vi "Auxiliary_data_to_file.vi"(2 "error in":errorcluster, 3 "Auxiliary Data":T1 {"EOS" items=["Ideal", "CH4_van_der_Waal", "CH4_Redlich_Kwong", "CO2_van_der_Waal", "CO2_Redlich_Kwong", ""]}, 4 "Byte Stream File in":refnum<file>) -> (0 "error out":errorcluster, 1 "Byte Stream File out":refnum<file>)   [LabVIEW 2016]
uses:
  auxiliary_cluster.ctl
  EOS.ctl
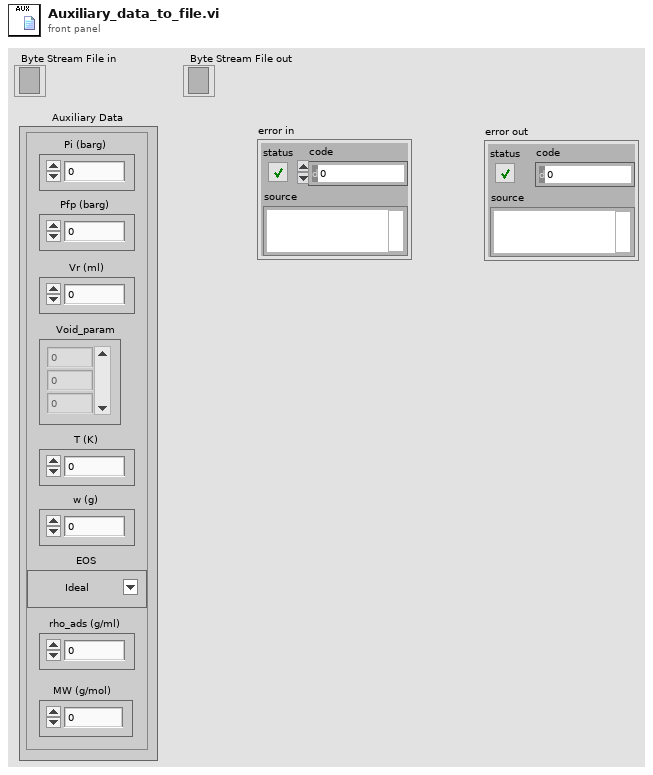
[diagram p1: front panel]
types:
  T1 = typedef "auxiliary_cluster.ctl" = cluster{"Pi (barg)":dbl, "Pfp (barg)":dbl, "Vr (ml)":dbl, "T (K)":dbl, "w (g)":dbl, "Void_param":dbl[], "EOS":T2, "rho_ads (g/ml)":dbl, "MW (g/mol)":dbl}
  T2 = typedef "EOS.ctl" = u16
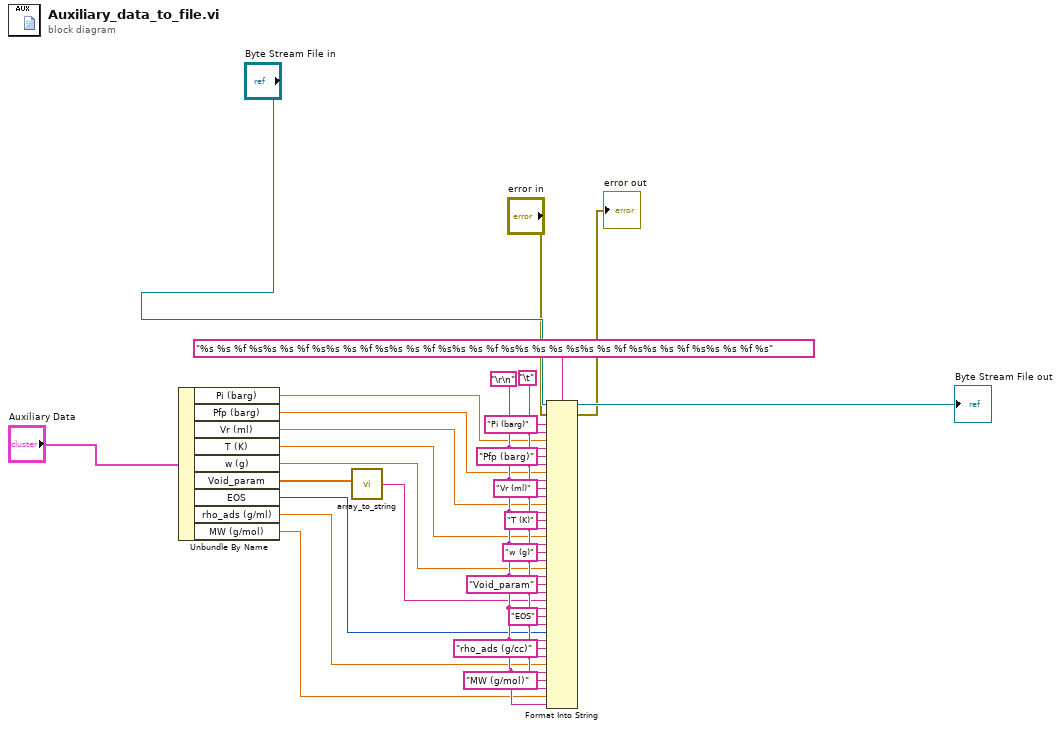
[diagram p0: block diagram]
diagram:
  w25 = "\r\n"
  w23 = "\t"
  n1 = Unbundle By Name("Auxiliary Data") -> ("Pi (barg)"=w14:dbl, "Pfp (barg)"=w15:dbl, "Vr (ml)"=w16:dbl, "T (K)"=w17:dbl, "w (g)"=w18:dbl, "Void_param"=w19:dbl[], "EOS"=w21:T2, "rho_ads (g/ml)"=w22:dbl, "MW (g/mol)"=w24:dbl)
  n2 = call "array_to_string.vi"("Void_param"=w19) -> ("String"=w20:string)
  n3 = Format Into String(format string="%s %s %f %s%s %s %f %s%s %s %f %s%s %s %f %s%s %s %f %s%s %s %s %s%s %s %f %s%s %s %f %s%s %s %f %s", initial string="Byte Stream File in", error in="error in", "Pi (barg)" ("input 1"), w23, w14, w25, "Pfp (barg)" ("input 5"), w23, w15, w25, "Vr (ml)" ("input 9"), w23, w16, w25, "T (K)" ("input 13"), w23, w17, w25, "w (g)" ("input 17"), w23, w18, w25, "Void_param" ("input 21"), w23, w20, w25, "EOS" ("input 25"), w23, w21, w25, "rho_ads (g/cc)" ("input 29"), w23, w22, w25, "MW (g/mol)" ("input 33"), w23, w24, w25) -> (resulting string=→"Byte Stream File out":refnum<file>, error out=→"error out":errorcluster)
